vi "main_ctrl.vi"(8 "error in":errorcluster) -> (0 "error out":errorcluster caption="Error")   [LabVIEW 2013]
uses:
  <vilib>/Rock Robotics/WPI/DriverStation/WPI_DriverStationRobotMode2.ctl
  typedefs/test/test data.ctl
  typedefs/test/test controls.ctl
  typedefs/fg_getset.ctl
  typedefs/vision/vision enable.ctl
  typedefs/vision/vision data.ctl
  typedefs/state machine/subStates.ctl
  typedefs/state machine/singleUseSubstate.ctl
  <vilib>/Rock Robotics/WPI/Solenoid/WPI_SolenoidValue.ctl
  <vilib>/Rock Robotics/WPI/Compressor/WPI_CompressorGetSetRefNum.vi
  <vilib>/Rock Robotics/WPI/RobotDrive/WPI_RobotDriveGetSetRefNum.vi
  <vilib>/Rock Robotics/WPI/RobotDrive/WPI_RobotDriveArcadeDrive_Standard(NoSaturation).vi
  <vilib>/Rock Robotics/WPI/Solenoid/WPI_SolenoidSetEnum.vi
panel:
  out "vision errors":errorcluster
  in  "Test\nControls":T1 {"Slider" scale=-1.0..1.0}
  out "Test Data":T2
  out "Robot Mode":T3
  out "Vision mSPI":u32
  out "Vision IPS":dbl
  out "Main IPS":dbl
  out "Main mSPI":u32
  # "Test Input/Output"
  # "MAIN CONTROL"
  # "holds robot control code - dual parallel state machine"
  # "SPI: milliseconds per iteration\nIPS: iterations per second"
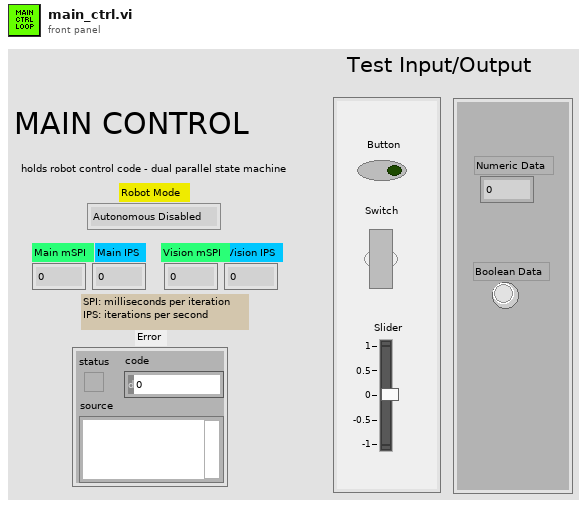
[diagram p1: front panel]
types:
  T1 = typedef "test controls.ctl" = cluster{"Button":bool, "Switch":bool, "Slider":dbl}
  T2 = typedef "test data.ctl" = cluster{"Numeric Data":dbl, "Boolean Data":bool}
  T3 = typedef "WPI_DriverStationRobotMode2.ctl" = enum16{"Autonomous Disabled", "Autonomous Enabled", "Teleop Disabled", "Teleop Enabled", "Timeout", "Finish", "Test Disabled", "Test Enabled"}
  T4 = typedef "fg_getset.ctl" = enum16{"Get", "Set"}
  T5 = typedef "vision data.ctl" = cluster{"x":dbl, "y":dbl, "area":dbl, "width":dbl, "height":dbl}
  T6 = typedef "vision enable.ctl" = enum16{"Enable", "Disable", "Stop"}
  T7 = typedef "WPI_CameraDevRef.ctl" = cluster{"Camera Address":string, "CameraStatus":errorcluster, "Acquire Image Notifier":refnum<notifier>}
  T8 = typedef "IMAQ Image.ctl" = refnum<image>
  T9 = cluster{"Vision mSPI":u32, "Main mSPI":u32, "Dash mSPI":u32}
  T10 = typedef "WPI_SolenoidDevRef.ctl" = cluster{"DevStatus":errorcluster, "Solenoid Module":T11, "Forward Solenoid Channel":T12, "Reverse Solenoid Channel":T12}
  T11 = typedef "FPGA_TypedefSolenoidModule.ctl" = enum16{"Solenoid Module 1", "Solenoid Module 2"}
  T12 = typedef "WPI_SolenoidChannel.ctl" = enum8{"Solenoid 1", "Solenoid 2", "Solenoid 3", "Solenoid 4", "Solenoid 5", "Solenoid 6", "Solenoid 7", "Solenoid 8", "Invalid"}
  T13 = typedef "WPI_RobotDriveDevRef.ctl" = cluster{"DevStatus":errorcluster, "Motors[]":T14[], "Square Inputs":bool, "Max Output":dbl, "Isochronous":bool}
  T14 = typedef "WPI_MotorControlDeviceRef.ctl" = cluster{"DeviceStatus":errorcluster, "Type":enum16{"PWM", "CAN"}, "PWM":cluster{"Digital Module":T15, "PWM Channel":T16, "DeadBand":T17}, "CAN":cluster{"Device Number":u8, "Control Mode":T18, "Semaphore":T19, "Max Vout":dbl}, "Invert":bool, "TransformRef":T20, "InvTransformRef":T20}
  T15 = typedef "FPGA_TypedefDigitalModule.ctl" = enum16{"Digital Module 1", "Digital Module 2"}
  T16 = typedef "FPGA_DIOPWMChannel.ctl" = enum8{"PWM 1", "PWM 2", "PWM 3", "PWM 4", "PWM 5", "PWM 6", "PWM 7", "PWM 8", "PWM 9", "PWM 10", "Invalid"}
  T17 = typedef "WPI_PWMDeadband.ctl" = cluster{"Name":string, "maxPositivePwm":i32, "minPositivePwm":i32, "centerPwm":i32, "maxNegativePwm":i32, "minNegativePwm":i32, "angularRange":u16}
  T18 = typedef "WPI_CANJaguar_ControlMode.ctl" = enum8{"Percent VBus", "Current", "Speed", "Position", "Voltage"}
  T19 = typedef "Semaphore RefNum" = refnum<k1>
  T20 = typedef "WPI_PWMTransform_ConPane.ctl" = refnum<vi>
  T21 = typedef "WPI_CompressorDevRef.ctl" = cluster{"DevStatus":errorcluster, "DigitalInputDevRef":T22, "RelayDevRef":T24}
  T22 = typedef "WPI_DigitalInputDevRef.ctl" = cluster{"DevStatus":errorcluster, "DIO Channel":T23, "Digital Module":T15}
  T23 = typedef "FPGA_DIOChannel.ctl" = enum8{"DIO 1", "DIO 2", "DIO 3", "DIO 4", "DIO 5", "DIO 6", "DIO 7", "DIO 8", "DIO 9", "DIO 10", "DIO 11", "DIO 12", "DIO 13", "DIO 14", "Invalid"}
  T24 = typedef "WPI_RelayDevRef.ctl" = cluster{"DevStatus":errorcluster, "Relay Channel":T25, "Digital Module":T15, "Relay Direction":T26}
  T25 = typedef "FPGA_DIORelayChannel.ctl" = enum8{"Relay 1", "Relay 2", "Relay 3", "Relay 4", "Relay 5", "Relay 6", "Relay 7", "Relay 8", "Invalid"}
  T26 = typedef "WPI_RelayDirection.ctl" = enum16{"Both directions", "Forward only", "Reverse only"}
  T27 = typedef "WPI_SolenoidValue.ctl" = enum16{"Off", "On", "Forward", "Reverse"}
  T28 = typedef "singleUseSubstate.ctl" = enum16{"null", "wait", "shift high", "shift low", "end"}
  T29 = typedef "WPI_DriverStationDerivedRobotMode.ctl" = enum16{"Init", "Execute", "Stop"}
  T30 = typedef "subStates.ctl" = enum16{"null", "wait", "driver control", "auto", "manual override", "hold position", "rotate", "test", "end"}
  T31 = typedef "Loop 2 Datatype.ctl" = cluster{"State":T30, "Waiting Loop":i32, "State to Wait For":i32, "Loop ID":i32, "Exit Value":i32}
  T32 = typedef "Loop 1 Datatype.ctl" = cluster{"State":T30, "Waiting Loop":i32, "State to Wait For":i32, "Loop ID":i32, "Exit Value":i32}
  T33 = typedef "Loop 3 Datatype.ctl" = cluster{"State":T30, "Waiting Loop":i32, "State to Wait For":i32, "Loop ID":i32, "Exit Value":i32}
  T34 = typedef "Loop 0 Datatype.ctl" = cluster{"State":T30, "Waiting Loop":i32, "State to Wait For":i32, "Loop ID":i32, "Exit Value":i32, "X Axis":dbl, "Y Axis":dbl, "Z Axis":dbl}
  T35 = typedef "Loop 4 Datatype.ctl" = cluster{"State":T30, "Waiting Loop":i32, "State to Wait For":i32, "Loop ID":i32, "Exit Value":i32}
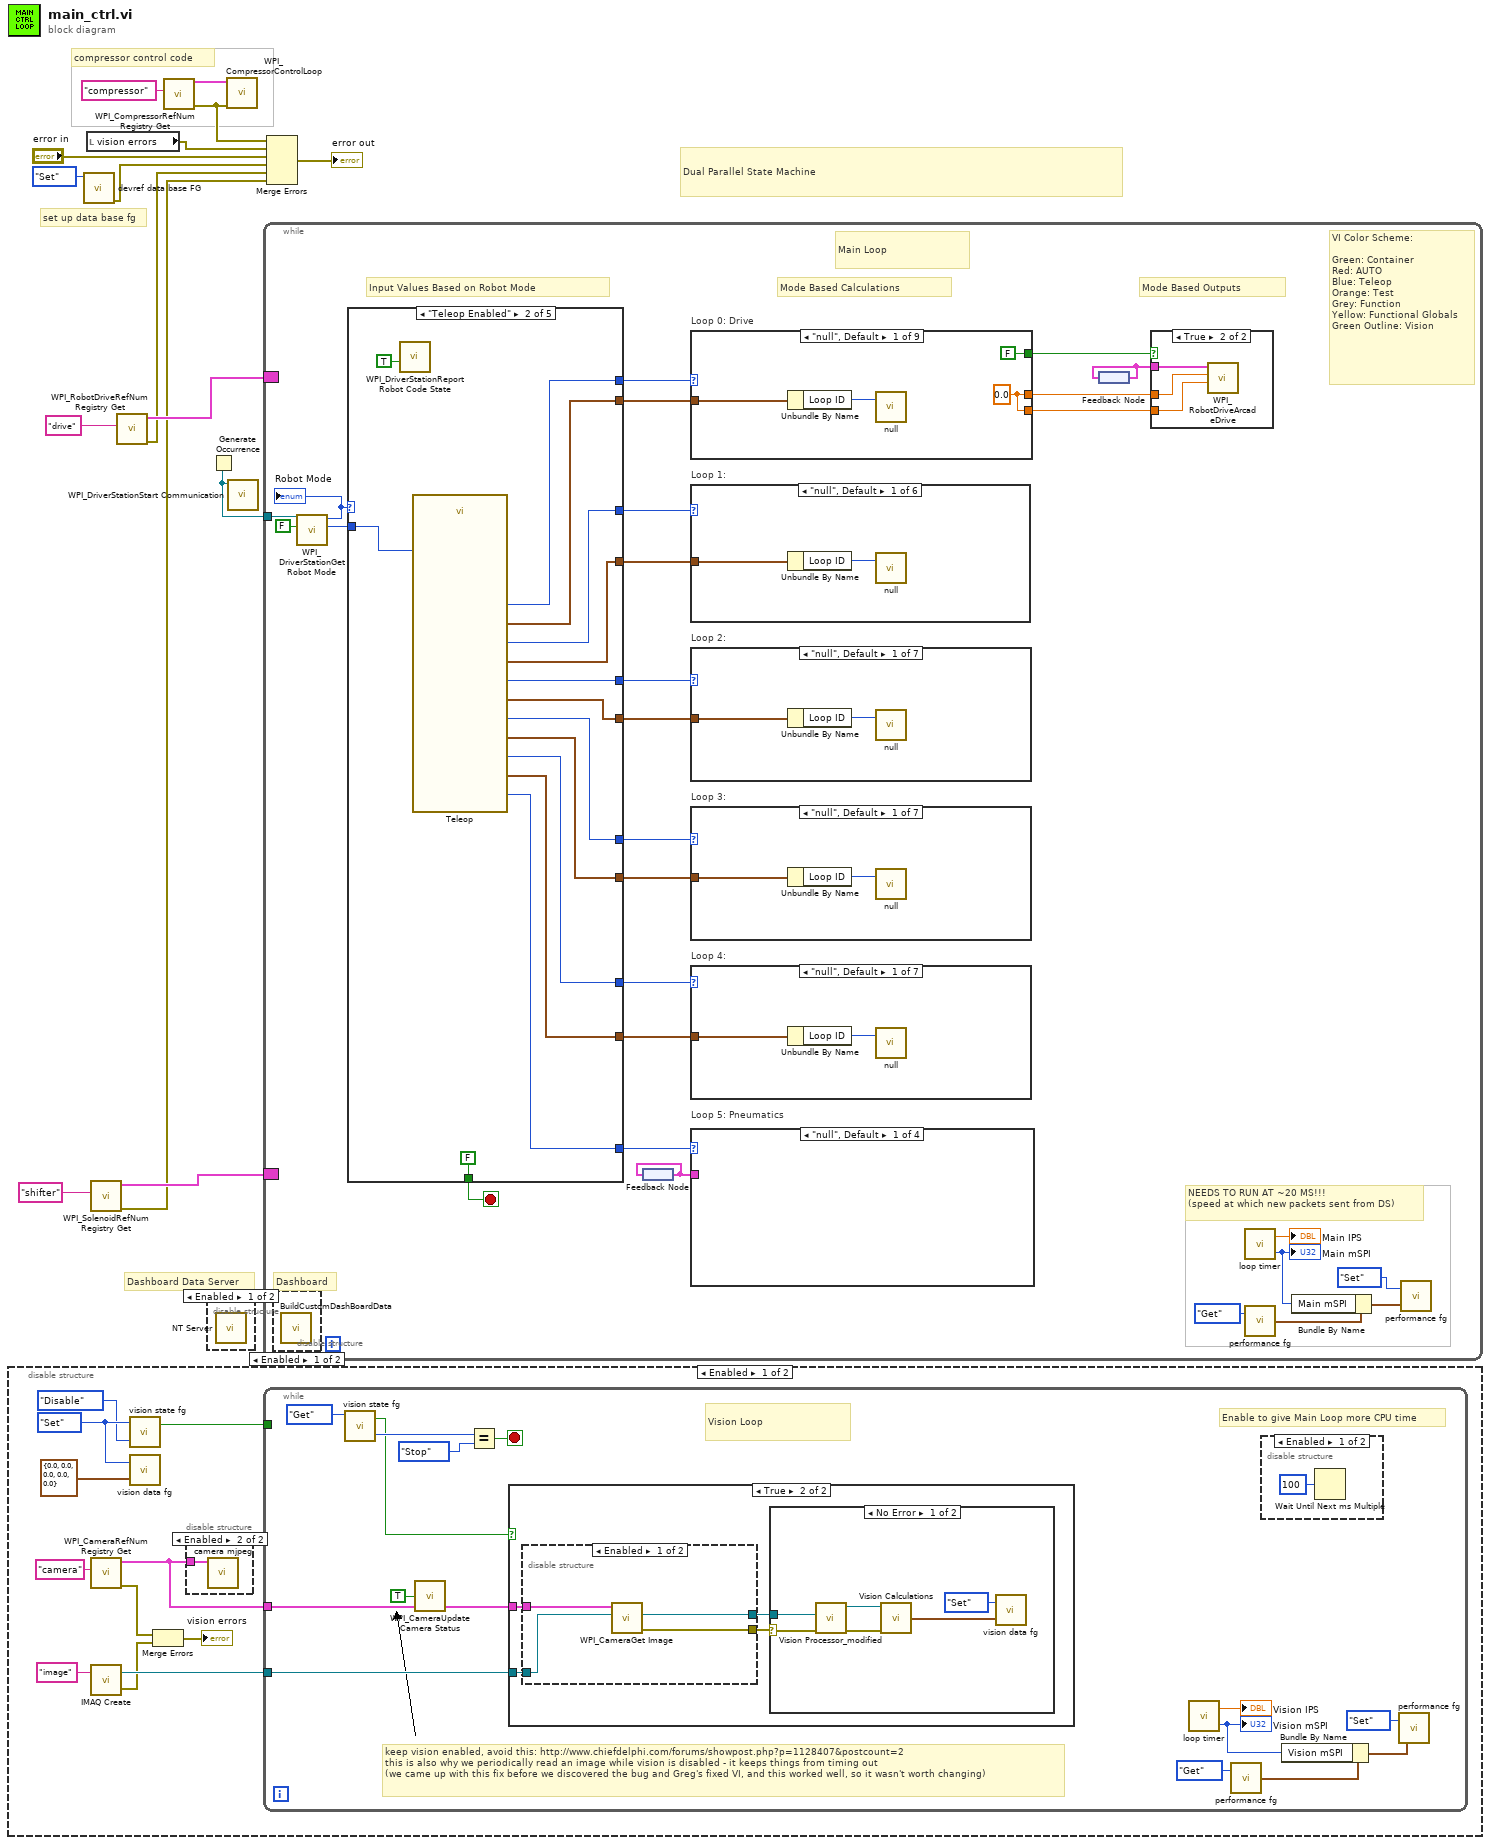
[diagram p0: block diagram]
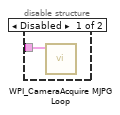
[diagram p3: hidden frame]
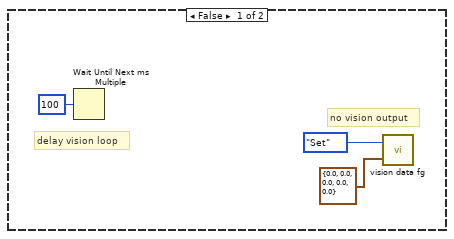
[diagram p5: hidden frame]
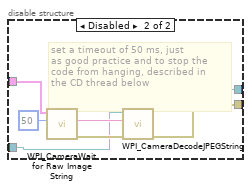
[diagram p7: hidden frame]
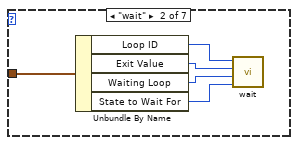
[diagram p9: hidden frame]
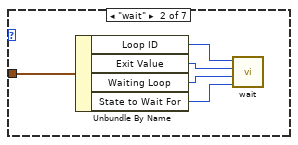
[diagram p15: hidden frame]
diagram:
  # "compressor control code"
  # "set up data base fg"
  # "Dual Parallel State Machine"
  # "Dashboard Data Server"
  n1 = disable-structure shown="Enabled" {
    frame Enabled {
      w24 = fg_getset."Set" ("Enum")
      n2 = call <vilib>:"WPI_CameraRefNum Registry Get.vi"("refnum name"="camera") -> ("error out"=w17:errorcluster, "CameraDevRef"=w21:T7)  [unwired: 9 in]
      n3 = call "IMAQ Create"("Image Name"="image") -> ("New Image"=w26:T8, "error out"=w18:errorcluster)  [unwired: 4 in]
      n4 = call "vision state fg.vi"("Action"=vision_enable."Disable", "Menu"=w24) -> ("Enabled?"=w25:bool)  [unwired: 1 out]
      n5 = call "vision data fg.vi"("Input"=T5 {"x"=0.0, "y"=0.0, "area"=0.0, "width"=0.0, "height"=0.0} ("Cluster"), "Menu"=w24) -> ()  [unwired: 1 out]
      n6 = Merge Errors(w17, w18) -> (→"vision errors":errorcluster)
      n7 = disable-structure shown="Enabled" {
        disable-tunnel: w21 -> [w27 w28]
        frame Disabled {
          n8 = call <vilib>:"WPI_CameraAcquire MJPG Loop.vi"("CameraDevRef"=w27) -> ()  [unwired: 11 in]
        }
        frame Enabled {
          n9 = call "camera mjpeg.vi"("CameraDevRef"=w28) -> ()  [unwired: 11 in]
        }
      }
      n10 = while {
        tunnel: w26 -> [w42]
        tunnel: w21 -> [w41]
        tunnel: w25 -> [_]
        stop <- w43 stop-if-true
        # "Enable to give Main Loop more CPU time"
        # "keep vision enabled, avoid this: http://www.chiefdelphi.com/forums/showpost.php?p=1128407&postcount=2\nthis is also why we periodically read an image while vision is disabled - it keeps things from timing out\n(we came up with this fix before we discovered the bug and Greg's fixed VI, and this worked well, so it wasn't worth changing)"
        # "Vision Loop"
        n11 = call "vision state fg.vi"("Menu"=fg_getset."Get" ("Enum")) -> ("State Out"=w37:T6, "Enabled?"=w29:bool)  [unwired: 1 in]
        n12 = call <vilib>:"WPI_CameraUpdate Camera Status.vi"("CameraDevRef In"=w41, "Enable Vision"=TRUE) -> ("CameraDevRef Out"=w40:T7)  [unwired: 3 in]
        n13 = Equal?(x=w37, y=vision_enable."Stop") -> (x = y?=w43:bool)
        n14 = case shown="True" w29 {
          tunnel: w42 -> [_ w51]
          tunnel: w40 -> [_ w50]
          frame False {
            # "no vision output"
            # "delay vision loop"
            n15 = Wait Until Next ms Multiple(millisecond multiple=u32 100) -> ()  [unwired: 1 out]
            n16 = call "vision data fg.vi"("Input"=T5 {"x"=0.0, "y"=0.0, "area"=0.0, "width"=0.0, "height"=0.0} ("Cluster"), "Menu"=fg_getset."Set" ("Enum")) -> ()  [unwired: 1 out]
          }
          frame True {
            n17 = disable-structure shown="Enabled" {
              disable-tunnel: w51 -> [w60 w64]
              disable-tunnel: w50 -> [w61 w66]
              disable-tunnel: [w59 w63] -> w49
              disable-tunnel: [w58 w62] -> w48
              frame Enabled {
                n18 = call <vilib>:"WPI_CameraGet Image.vi"("Image"=w60, "CameraDevRef"=w61) -> ("error out"=w58:errorcluster, "Image Out"=w59:T8)  [unwired: 7 in, 1 out]
              }
              frame Disabled {
                # "set a timeout of 50 ms, just\nas good practice and to stop the \ncode from hanging, described in \nthe CD thread below"
                n19 = call <vilib>:"WPI_CameraWait for Raw Image String.vi"("Timeout in ms (-1)"=50, "CameraDevRef"=w66) -> ("error out"=w68:errorcluster, "String"=w67:string)  [unwired: 3 in, 5 out]
                n20 = call <vilib>:"WPI_CameraDecodeJPEGString.vi"("error in"=w68, "Compressed Image"=w67, "Image In"=w64) -> ("error out"=w62:errorcluster, "Image Out"=w63:T8)  [unwired: 3 out]
              }
            }
            n21 = case shown="No Error" w48 {
              selector: w48 -> [w56 _]
              tunnel: w49 -> [w55 _]
              frame No Error {
                n22 = call "Vision Processor_modified.vi"("error in"=w56, "Image In"=w55) -> ("error out"=w53:errorcluster, "Image Out"=w54:T8)  [unwired: 5 in]
                n23 = call "Vision Calculations.vi"("Image In"=w54, "error in"=w53) -> ("Vision Data"=w52:T5)  [unwired: 3 in]
                n24 = call "vision data fg.vi"("Input"=w52, "Menu"=fg_getset."Set" ("Enum")) -> ()  [unwired: 1 out]
              }
              frame Error {
              }
            }
          }
        }
        n25 = call "loop timer.vi"() -> ("IPS"=→"Vision IPS":dbl, "SPI"=w35:u32)  [unwired: 1 in]
        "Vision mSPI" <- w35
        n26 = call "performance fg.vi"("Menu"=fg_getset."Get") -> ("Output"=w33:T9)  [unwired: 1 in]
        n27 = disable-structure shown="Enabled" {
          frame Enabled {
            n28 = Wait Until Next ms Multiple(millisecond multiple=u32 100) -> ()  [unwired: 1 out]
          }
          frame Disabled {
          }
        }
        n29 = Bundle By Name(cluster=w33, "Vision mSPI"=w35) -> (w32:T9)
        n30 = call "performance fg.vi"("Input"=w32, "Menu"=fg_getset."Set") -> ()  [unwired: 1 out]
      }
    }
    frame Disabled {
      # "vision disabled"
    }
  }
  n31 = call "devref data base FG.vi"("Menu"=fg_getset."Set") -> ("error out"=w3:errorcluster)  [unwired: 5 in, 5 out]
  n32 = local read "vision errors"() -> (w5:errorcluster)
  n33 = call <vilib>:"WPI_SolenoidRefNum Registry Get.vi"("refnum name"="shifter") -> ("error out"=w1:errorcluster, "SolenoidDevRef"=w11:T10)  [unwired: 9 in]
  n34 = call <vilib>:"WPI_RobotDriveRefNum Registry Get.vi"("refnum name"="drive") -> ("error out"=w2:errorcluster, "RobotDriveDevRef"=w7:T13)  [unwired: 9 in]
  n35 = call <vilib>:"WPI_CompressorRefNum Registry Get.vi"("refnum name"="compressor") -> ("error out"=w6:errorcluster, "CompressorDevRef"=w12:T21)  [unwired: 9 in]
  n36 = disable-structure shown="Enabled" {
    frame Enabled {
      n37 = call <vilib>:"NT Server.vi"() -> ()  [unwired: 12 in]
    }
    frame Disabled {
    }
  }
  n38 = Generate Occurrence() -> (w9:refnum<k4>)
  n39 = call <vilib>:"WPI_CompressorControlLoop.vi"("error in (no error)"=w6, "CompressorDevRef"=w12) -> ()  [unwired: 10 in]
  n40 = call <vilib>:"WPI_DriverStationStart Communication.vi"("occurrence"=w9) -> ()  [unwired: 11 in]
  n41 = while {
    tunnel: w9 -> [w78]
    border: w7 -> [_]
    border: w11 -> [_]
    stop <- w92 stop-if-true
    # "Dashboard"
    # "Mode Based Outputs"
    # "VI Color Scheme:\n\nGreen: Container\nRed: AUTO\nBlue: Teleop\nOrange: Test \nGrey: Function\nYellow: Functional Globals\nGreen Outline: Vision"
    # "Input Values Based on Robot Mode"
    # "Mode Based Calculations"
    # "NEEDS TO RUN AT ~20 MS!!!\n(speed at which new packets sent from DS)"
    # "Main Loop"
    n42 = disable-structure shown="Enabled" {
      frame Enabled {
        n43 = call "BuildCustomDashBoardData.vi"() -> ()  [unwired: 12 in]
      }
      frame Disabled {
      }
    }
    n44 = call <vilib>:"WPI_DriverStationGet Robot Mode.vi"("Finish"=FALSE, "DS Occurrence"=w78) -> ("Call Context"=w77:T29, "Robot Mode"=w76:T3)  [unwired: 8 out]
    "Robot Mode" <- w76
    n45 = case shown="\"Teleop Enabled\"" w76 {
      tunnel: [w188 w205 w217 w222 w228] -> w80
      tunnel: w77 -> [w181 w201 w208 _ _]
      tunnel: [w186 w204 w219 w222 w228] -> w94
      tunnel: [w182 w202 w211 singleUseSubstate."null" ("SubState 5") singleUseSubstate."end" ("SubState 5")] -> w93
      tunnel: [FALSE FALSE FALSE FALSE TRUE] -> w92
      tunnel: [w190 w200 w215 w222 w228] -> w75
      tunnel: [w189 w199 w216 _ _] -> w86
      tunnel: [w187 w198 w218 _ _] -> w85
      tunnel: [w185 w197 w214 _ _] -> w84
      tunnel: [w183 w196 w212 _ _] -> w71
      tunnel: [w184 w195 w213 w222 w228] -> w72
      tunnel: [w178 w193 w206 _ _] -> w69
      tunnel: [w179 w192 w207 w222 w228] -> w70
      frame "Autonomous Enabled" {
        n46 = call <vilib>:"WPI_DriverStationReport Robot Code State.vi"("Autonomous"=TRUE) -> ()  [unwired: 10 in, 1 out]
        n47 = call "Autonomous.vi"("Call Context"=w181) -> ("SubState 2"=w186:T30, "Loop 2 Data"=w185:T31, "SubState 1"=w188:T30, "Loop 1 Data"=w187:T32, "Loop 3 Data"=w183:T33, "SubState 0"=w190:T30, "SubState 3"=w184:T30, "Loop 0 Data"=w189:T34, "SubState 4"=w179:T30, "Loop 4 Data"=w178:T35, "SubState 5"=w182:T28)
      }
      frame "Teleop Enabled" {
        n48 = call <vilib>:"WPI_DriverStationReport Robot Code State.vi"("TeleOp"=TRUE) -> ()  [unwired: 10 in, 1 out]
        n49 = call "Teleop.vi"("Call Context"=w201) -> ("SubState 3"=w195:T30, "SubState 4"=w192:T30, "SubState 5"=w202:T28, "Loop 4 Data"=w193:T35, "Loop 3 Data"=w196:T33, "SubState 0"=w200:T30, "Loop 1 Data"=w198:T32, "Loop 0 Data"=w199:T34, "SubState 1"=w205:T30, "Loop 2 Data"=w197:T31, "SubState 2"=w204:T30)  [unwired: 8 in]
      }
      frame "Test Enabled" {
        n50 = call "test io.vi"("Call Context"=w208) -> ("Test Data"=→"Test Data":T2)
        n51 = call <vilib>:"WPI_DriverStationReport Robot Code State.vi"("Test"=TRUE) -> ()  [unwired: 10 in, 1 out]
        n52 = call "Test.vi"("Call Context"=w208, "Test Controls"="Test\nControls") -> ("SubState 0"=w215:T30, "SubState 4"=w207:T30, "Loop 0 Data"=w216:T34, "SubState 1"=w217:T30, "Loop 1 Data"=w218:T32, "SubState 2"=w219:T30, "SubState 5"=w211:T28, "Loop 3 Data"=w212:T33, "Loop 4 Data"=w206:T35, "SubState 3"=w213:T30, "Loop 2 Data"=w214:T31)  [unwired: 3 in]
      }
      frame "Autonomous Disabled", "Teleop Disabled", "Timeout", "Test Disabled" {
        w222 = subStates."null" ("SubState 0")
        # "set all loops to null"
        # "make sure to disable vision\nwe don't need it here"
        # "Robot Disabled, Timeout"
        n53 = call <vilib>:"WPI_DriverStationReport Robot Code State.vi"("Disabled"=TRUE) -> ()  [unwired: 10 in, 1 out]
        n54 = call "vision state fg.vi"("Action"=vision_enable."Disable", "Menu"=fg_getset."Set") -> ()  [unwired: 2 out]
      }
      frame "Finish" {
        w228 = subStates."end" ("Loop State")
        # "Stop DS Comms"
        # "stop vision loop"
        # "Stop All Loops"
        # "stop the while loop"
        n55 = call <vilib>:"WPI_DriverStationStop Communication.vi"("StopCommunication"=TRUE) -> ()  [unwired: 10 in, 1 out]
        n56 = call "vision state fg.vi"("Action"=vision_enable."Stop", "Menu"=fg_getset."Set") -> ()  [unwired: 2 out]
      }
    }
    n57 = feedback #1() -> (w83:T10)
    n58 = feedback-in #1(w83) -> ()
    n59 = case "Loop 0: Drive" shown="\"null\", Default" w75 {
      tunnel: w86 -> [w126 w129 w137 w143 w151 w153 w160 _ _]
      tunnel: [w125 w128 w136 w140 w148 w155 w162 w163 w166] -> w74
      tunnel: [w125 w128 w135 w139 w147 w154 w161 w163 w166] -> w73
      tunnel: [FALSE FALSE TRUE FALSE FALSE FALSE FALSE TRUE FALSE] -> w82
      frame "null", Default {
        w125 = 0.0 ("X Axis")
        n60 = Unbundle By Name(w126) -> ("Loop ID"=w123:i32)
        n61 = call "null.vi"("This Loop ID"=w123) -> ()  [unwired: 2 in]
      }
      frame "wait" {
        w128 = 0.0 ("X Axis")
        n62 = Unbundle By Name(w129) -> ("Loop ID"=w133:i32, "Exit Value"=w132:i32, "Waiting Loop"=w131:i32, "State to Wait For"=w130:i32)
        n63 = call "wait.vi"("State to wait for"=w130, "Waiting Loop ID"=w131, "Time (ms)"=w132, "Current Loop ID"=w133) -> ()  [unwired: 1 out]
      }
      frame "driver control" {
        n64 = Unbundle By Name(w137) -> ("X Axis"=w136:dbl, "Y Axis"=w135:dbl)
      }
      frame "manual override" {
        n65 = Unbundle By Name(w143) -> ("X Axis"=w142:dbl, "Y Axis"=w141:dbl)
        n66 = expression code="x/2"(w142) -> (w140:dbl)
        n67 = expression code="x/2"(w141) -> (w139:dbl)
      }
      frame "hold position" {
        n68 = Unbundle By Name(w151) -> ("X Axis"=w150:dbl, "Y Axis"=w149:dbl)
        n69 = call "closed hold.vi"("Acrade Drive?"=TRUE, "Y axis value (Left)"=w149, "X axis value (Right)"=w150, "Threshold (.4)"=0.4) -> ("right"=w147:dbl, "left"=w148:dbl)
      }
      frame "auto" {
        n70 = Unbundle By Name(w153) -> ("X Axis"=w152:dbl)
        n71 = call "autoDrive.vi"("Distance"=w152) -> ("right speed"=w154:dbl, "left speed"=w155:dbl)  [unwired: 2 in, 1 out]
      }
      frame "rotate" {
        n72 = Unbundle By Name(w160) -> ("X Axis"=w159:dbl, "Y Axis"=w158:dbl)
        n73 = call "rotate.vi"("Rate"=w158, "Angle"=w159) -> ("right speed"=w161:dbl, "left speed"=w162:dbl)  [unwired: 1 in, 1 out]
      }
      frame "test" {
        w163 = 0.0
      }
      frame "end" {
        w166 = 0.0 ("X Axis")
      }
    }
    n74 = case "Loop 1:" shown="\"null\", Default" w80 {
      tunnel: w85 -> [w172 w173 _ _ _ _]
      frame "null", Default {
        n75 = Unbundle By Name(w172) -> ("Loop ID"=w171:i32)
        n76 = call "null.vi"("This Loop ID"=w171) -> ()  [unwired: 2 in]
      }
      frame "wait" {
        n77 = Unbundle By Name(w173) -> ("Loop ID"=w177:i32, "Exit Value"=w176:i32, "Waiting Loop"=w175:i32, "State to Wait For"=w174:i32)
        n78 = call "wait.vi"("State to wait for"=w174, "Waiting Loop ID"=w175, "Time (ms)"=w176, "Current Loop ID"=w177) -> ()  [unwired: 1 out]
      }
      frame "auto" {
      }
      frame "manual override" {
      }
      frame "test" {
      }
      frame "end" {
      }
    }
    n79 = case "Loop 2:" shown="\"null\", Default" w94 {
      tunnel: w84 -> [w111 w112 _ _ _ _ _]
      frame "null", Default {
        n80 = Unbundle By Name(w111) -> ("Loop ID"=w110:i32)
        n81 = call "null.vi"("This Loop ID"=w110) -> ()  [unwired: 2 in]
      }
      frame "wait" {
        n82 = Unbundle By Name(w112) -> ("Loop ID"=w116:i32, "Exit Value"=w115:i32, "Waiting Loop"=w114:i32, "State to Wait For"=w113:i32)
        n83 = call "wait.vi"("State to wait for"=w113, "Waiting Loop ID"=w114, "Time (ms)"=w115, "Current Loop ID"=w116) -> ()  [unwired: 1 out]
      }
      frame "driver control" {
      }
      frame "manual override" {
      }
      frame "auto" {
      }
      frame "test" {
      }
      frame "end" {
      }
    }
    n84 = case "Loop 3:" shown="\"null\", Default" w72 {
      tunnel: w71 -> [w104 w105 _ _ _ _ _]
      frame "null", Default {
        n85 = Unbundle By Name(w104) -> ("Loop ID"=w103:i32)
        n86 = call "null.vi"("This Loop ID"=w103) -> ()  [unwired: 2 in]
      }
      frame "wait" {
        n87 = Unbundle By Name(w105) -> ("Loop ID"=w109:i32, "Exit Value"=w108:i32, "Waiting Loop"=w107:i32, "State to Wait For"=w106:i32)
        n88 = call "wait.vi"("State to wait for"=w106, "Waiting Loop ID"=w107, "Time (ms)"=w108, "Current Loop ID"=w109) -> ()  [unwired: 1 out]
      }
      frame "driver control" {
      }
      frame "manual override" {
      }
      frame "auto" {
      }
      frame "test" {
      }
      frame "end" {
      }
    }
    n89 = case "Loop 4:" shown="\"null\", Default" w70 {
      tunnel: w69 -> [w97 w98 _ _ _ _ _]
      frame "null", Default {
        n90 = Unbundle By Name(w97) -> ("Loop ID"=w96:i32)
        n91 = call "null.vi"("This Loop ID"=w96) -> ()  [unwired: 2 in]
      }
      frame "wait" {
        n92 = Unbundle By Name(w98) -> ("Loop ID"=w102:i32, "Exit Value"=w101:i32, "Waiting Loop"=w100:i32, "State to Wait For"=w99:i32)
        n93 = call "wait.vi"("State to wait for"=w99, "Waiting Loop ID"=w100, "Time (ms)"=w101, "Current Loop ID"=w102) -> ()  [unwired: 1 out]
      }
      frame "driver control" {
      }
      frame "manual override" {
      }
      frame "auto" {
      }
      frame "test" {
      }
      frame "end" {
      }
    }
    n94 = case "Loop 5: Pneumatics" shown="\"null\", Default" w93 {
      tunnel: w83 -> [_ _ w168 w169]
      frame "null", Default {
      }
      frame "wait" {
      }
      frame "shift high" {
        n95 = call-poly <vilib>:"WPI_SolenoidSet.vi"("Value"=WPI_SolenoidValue."Forward", "SolenoidDevRef"=w168) -> ()  [unwired: 8 in, 2 out]
      }
      frame "shift low" {
        n96 = call-poly <vilib>:"WPI_SolenoidSet.vi"("Value"=WPI_SolenoidValue."Reverse", "SolenoidDevRef"=w169) -> ()  [unwired: 8 in, 2 out]
      }
    }
    n97 = feedback #2() -> (w81:T13)
    n98 = feedback-in #2(w81) -> ()
    n99 = case shown="True" w82 {
      tunnel: w74 -> [w118 w122]
      tunnel: w73 -> [w117 w121]
      tunnel: w81 -> [w119 w120]
      frame False {
        n100 = call <vilib>:"WPI_RobotDriveMotors.vi"("RightSpeed"=w117, "LeftSpeed"=w118, "RobotDriveDevRef"=w119) -> ()  [unwired: 6 in, 3 out]
      }
      frame True {
        n101 = call-poly <vilib>:"WPI_RobotDriveArcadeDrive.vi"("Y axis value"=w121, "X axis value"=w122, "RobotDriveDevRef"=w120) -> ()  [unwired: 6 in, 3 out]
      }
    }
    n102 = call "loop timer.vi"() -> ("IPS"=→"Main IPS":dbl, "SPI"=w91:u32)  [unwired: 1 in]
    "Main mSPI" <- w91
    n103 = call "performance fg.vi"("Menu"=fg_getset."Get") -> ("Output"=w88:T9)  [unwired: 1 in]
    n104 = Bundle By Name(cluster=w88, "Main mSPI"=w91) -> (w87:T9)
    n105 = call "performance fg.vi"("Input"=w87, "Menu"=fg_getset."Set") -> ()  [unwired: 1 out]
  }
  n106 = Merge Errors(w6, w5, "error in", w3, w2, w1) -> (→"error out":errorcluster)
